vi "extract channel history.vi"(0 "Vmon Hist in":dbl[][](array[numeric]), 1 "Vset Hist in":dbl[][](array[numeric]), 2 "Imon Hist in":dbl[][](array[numeric]), 3 "Iset Hist in":dbl[][](array[numeric]), 4 "TS History":dbl[][](array[numeric]), 5 "index":i32) -> (7 "Vmon Hist out":dbl[](array[numeric]), 9 "Vset Hist out":dbl[](array[numeric]), 11 "Imon Hist out":dbl[](array[numeric]), 13 "Iset Hist out":dbl[](array[numeric]), 14 "Voltage":cluster{dbl[], dbl[]}[](array[cluster]), 19 "Current":cluster{dbl[], dbl[]}[](array[cluster]))   [LabVIEW 2018]
uses:
  <userlib>/_OpenG.lib/array/array.llb/Search 1D Array (DBL)__ogtk.vi
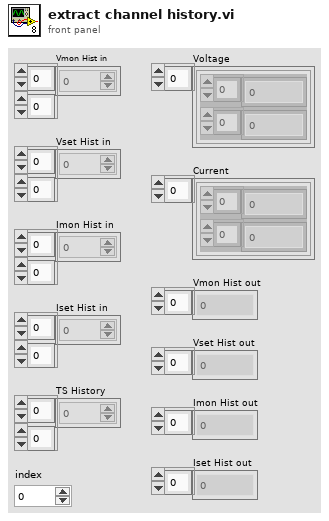
[diagram p1: front panel]
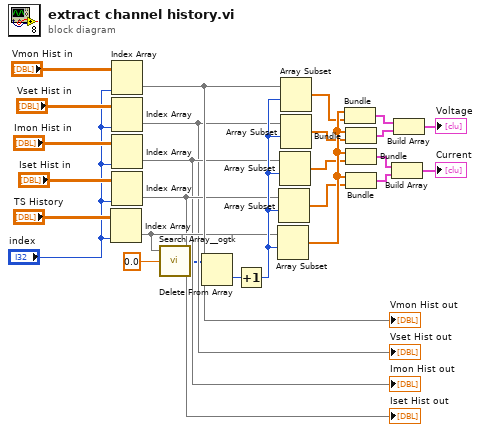
[diagram p0: block diagram]
diagram:
  n1 = Index Array(array="TS History", index (col)="index") -> (element=w16:dbl[])  [unwired: 1 in]
  n2 = Index Array(array="Vmon Hist in", index (col)="index") -> (element=w20:dbl[])  [unwired: 1 in]
  "Vmon Hist out" <- w20
  n3 = Index Array(array="Vset Hist in", index (col)="index") -> (element=w10:dbl[])  [unwired: 1 in]
  "Vset Hist out" <- w10
  n4 = Index Array(array="Imon Hist in", index (col)="index") -> (element=w12:dbl[])  [unwired: 1 in]
  "Imon Hist out" <- w12
  n5 = Index Array(array="Iset Hist in", index (col)="index") -> (element=w14:dbl[])  [unwired: 1 in]
  "Iset Hist out" <- w14
  n6 = call-poly <userlib>:"Search Array__ogtk.vi"("Array"=w16, "Element Data"=0.0 ("disabled index (col)")) -> ("Indices of Elements"=w7:i32[])  [unwired: 7 in]
  n7 = Delete From Array(array=w7) -> (deleted portion=w8:i32)  [unwired: 2 in, 1 out]
  n8 = Increment(x=w8) -> (x+1=w17:i32)
  n9 = Array Subset(array=w16, index=w17) -> (w26:dbl[])  [unwired: 1 in]
  n10 = Array Subset(array=w14, index=w17) -> (w15:dbl[])  [unwired: 1 in]
  n11 = Array Subset(array=w12, index=w17) -> (w13:dbl[])  [unwired: 1 in]
  n12 = Array Subset(array=w20, index=w17) -> (w9:dbl[])  [unwired: 1 in]
  n13 = Array Subset(array=w10, index=w17) -> (w11:dbl[])  [unwired: 1 in]
  n14 = Bundle(w26, w9) -> (w3:cluster{dbl[], dbl[]})  [unwired: 1 in]
  n15 = Bundle(w26, w11) -> (w4:cluster{dbl[], dbl[]})  [unwired: 1 in]
  n16 = Bundle(w26, w13) -> (w18:cluster{dbl[], dbl[]})  [unwired: 1 in]
  n17 = Bundle(w26, w15) -> (w19:cluster{dbl[], dbl[]})  [unwired: 1 in]
  n18 = Build Array(w18, w19) -> (→"Current":cluster{dbl[], dbl[]}[])
  n19 = Build Array(w3, w4) -> (→"Voltage":cluster{dbl[], dbl[]}[])
